vi "PicoScopeVoltsToAdc.vi"(0 "Max_adc":i16=32767, 1 "Volts":dbl, 2 "Range Index":u16) -> (3 "ADC count":i16)   [LabVIEW 2020]
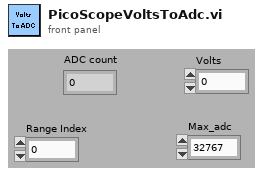
[diagram p1: front panel]
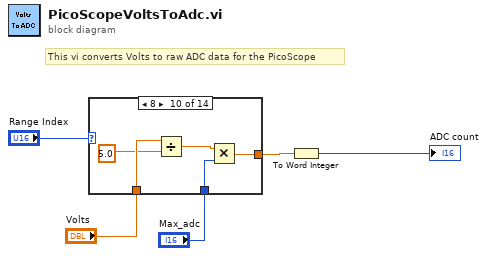
[diagram p0: block diagram]
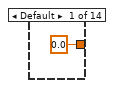
[diagram p2: hidden frame]
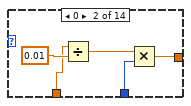
[diagram p3: hidden frame]
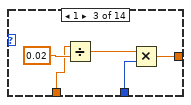
[diagram p4: hidden frame]
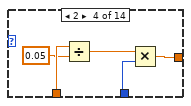
[diagram p5: hidden frame]
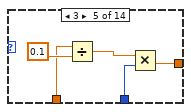
[diagram p6: hidden frame]
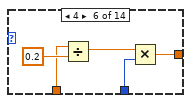
[diagram p7: hidden frame]
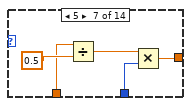
[diagram p8: hidden frame]
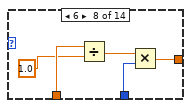
[diagram p9: hidden frame]
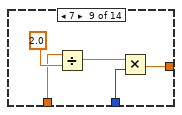
[diagram p10: hidden frame]
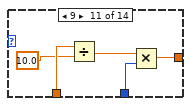
[diagram p11: hidden frame]
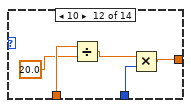
[diagram p12: hidden frame]
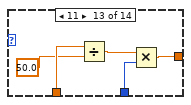
[diagram p13: hidden frame]
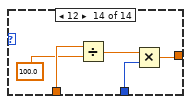
[diagram p14: hidden frame]
diagram:
  # "This vi converts Volts to raw ADC data for the PicoScope"
  n1 = case shown="8" "Range Index" {
    tunnel: [0.0 w9 w13 w21 w24 w31 w36 w41 w46 w51 w56 w61 w66 w67] -> w2
    tunnel: "Max_adc" -> [_ w8 w12 w18 w22 w30 w35 w40 w45 w50 w55 w60 w65 w69]
    tunnel: "Volts" -> [_ w7 w14 w20 w25 w27 w33 w38 w42 w49 w53 w58 w63 w71]
    frame Default {
    }
    frame 0 {
      n2 = Divide(x=w7, y=0.01 ("x")) -> (x/y=w11:dbl)
      n3 = Multiply(x=w11, y=w8) -> (x*y=w9:dbl)
    }
    frame 1 {
      n4 = Divide(x=w14, y=0.02 ("x")) -> (x/y=w16:dbl)
      n5 = Multiply(x=w16, y=w12) -> (x*y=w13:dbl)
    }
    frame 2 {
      n6 = Divide(x=w20, y=0.05 ("x")) -> (x/y=w17:dbl)
      n7 = Multiply(x=w17, y=w18) -> (x*y=w21:dbl)
    }
    frame 3 {
      n8 = Divide(x=w25, y=0.1 ("x")) -> (x/y=w23:dbl)
      n9 = Multiply(x=w23, y=w22) -> (x*y=w24:dbl)
    }
    frame 4 {
      n10 = Divide(x=w27, y=0.2 ("x")) -> (x/y=w29:dbl)
      n11 = Multiply(x=w29, y=w30) -> (x*y=w31:dbl)
    }
    frame 5 {
      n12 = Divide(x=w33, y=0.5 ("x")) -> (x/y=w32:dbl)
      n13 = Multiply(x=w32, y=w35) -> (x*y=w36:dbl)
    }
    frame 6 {
      n14 = Divide(x=w38, y=1.0 ("x")) -> (x/y=w39:dbl)
      n15 = Multiply(x=w39, y=w40) -> (x*y=w41:dbl)
    }
    frame 7 {
      n16 = Divide(x=w42, y=2.0 ("x")) -> (x/y=w44:dbl)
      n17 = Multiply(x=w44, y=w45) -> (x*y=w46:dbl)
    }
    frame 8 {
      n18 = Divide(x=w49, y=5.0 ("x")) -> (x/y=w47:dbl)
      n19 = Multiply(x=w47, y=w50) -> (x*y=w51:dbl)
    }
    frame 9 {
      n20 = Divide(x=w53, y=10.0 ("x")) -> (x/y=w54:dbl)
      n21 = Multiply(x=w54, y=w55) -> (x*y=w56:dbl)
    }
    frame 10 {
      n22 = Divide(x=w58, y=20.0 ("x")) -> (x/y=w59:dbl)
      n23 = Multiply(x=w59, y=w60) -> (x*y=w61:dbl)
    }
    frame 11 {
      n24 = Divide(x=w63, y=50.0 ("x")) -> (x/y=w64:dbl)
      n25 = Multiply(x=w64, y=w65) -> (x*y=w66:dbl)
    }
    frame 12 {
      n26 = Divide(x=w71, y=100.0 ("x")) -> (x/y=w68:dbl)
      n27 = Multiply(x=w68, y=w69) -> (x*y=w67:dbl)
    }
  }
  n28 = To Word Integer(number=w2) -> (16bit integer=→"ADC count":i16)
